vi "Read Timestamp.vi"(11 "Timestamp Event in":refnum<class "Timestamp Event.lvclass">) -> (2 "Timestamp":timestamp, 3 "Timestamp Event out":refnum<class "Timestamp Event.lvclass">)   [LabVIEW 2015, in "Example Source.lvlib" / "Timestamp Event.lvclass"]
uses:
  Timestamp Event.lvclass
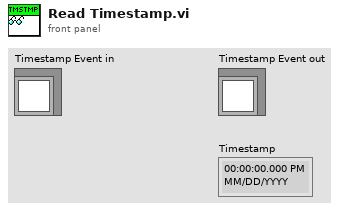
[diagram p1: front panel]
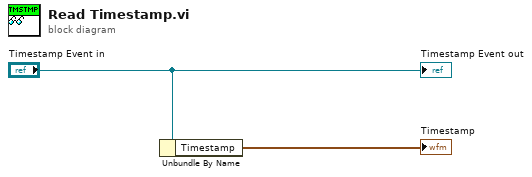
[diagram p0: block diagram]
diagram:
  n1 = Unbundle By Name("Timestamp Event in") -> ("Timestamp"=→"Timestamp":timestamp)
  "Timestamp Event out" <- "Timestamp Event in"
